vi "Close.vi"(8 "Error In":errorcluster, 11 "SFTP Directory":refnum<class "SFTP Directory.lvclass">) -> (0 "Error Out":errorcluster, 2 "Remote Path":string, 3 "SFTP":refnum<class "SFTP.lvclass">)   [LabVIEW 2018, in "Toolkit.lvlib" / "SFTP Directory.lvclass"]
uses:
  SFTP Directory.lvclass
  SFTP/SFTP.lvclass
  SFTP Directory.lvclass/SFTP Directory.ctl
  SFTP/SFTP.lvclass/SFTP.ctl
  Session/Session.lvclass/Session.ctl
  SSH/SSH.lvclass/SSH.ctl
  Toolkit.lvlib
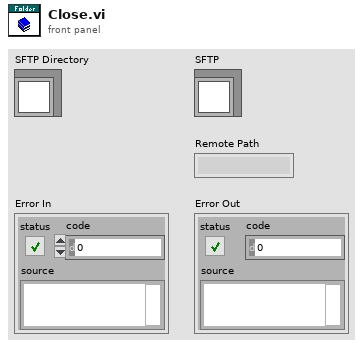
[diagram p1: front panel]
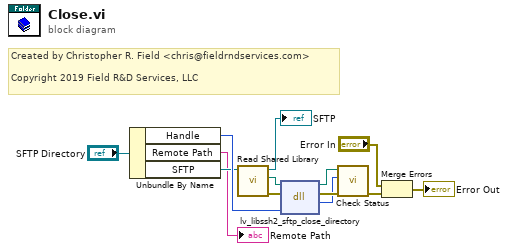
[diagram p0: block diagram]
diagram:
  # "Created by Christopher R. Field <chris@fieldrndservices.com>\n\nCopyright 2019 Field R&D Services, LLC"
  n1 = Unbundle By Name("SFTP Directory") -> ("Handle"=w11:u64, "Remote Path"=→"Remote Path":string, "SFTP"=w5:refnum<class "SFTP.lvclass">)
  n2 = call "Read Shared Library.vi"("SFTP In"=w5) -> ("Erorr Out"=w2:errorcluster, "libssh2lv Shared Library"=w3:path, "SFTP Out"=→"SFTP":refnum<class "SFTP.lvclass">)  [unwired: 8 in]
  n3 = dll-call lib="lv-libssh2.*" fn="lv_libssh2_sftp_close_directory"(path in=w3, error in=w2, "handle"=w11) -> (path out=w9:path, error out=w10:errorcluster, "status"=w7:i32)  [unwired: 2 in]
  n4 = call "Check Status.vi"("Error In"=w10, "Status"=w7, "lv-libssh2 Shared Library In"=w9) -> ("Error Out"=w8:errorcluster)  [unwired: 7 in, 1 out]
  n5 = Merge Errors("Error In", w8) -> (→"Error Out":errorcluster)
